vi "PH_Stepmotor_BaseClass.PC set Settings.vi"(0 "i ref in":refnum<vi>, 1 "axis":i32=-1, 2 "Settings to set":T1={"Sign change"=FALSE, "Width"=0.0, "Calibration"=0.0, "Unit"="Steps", "Motor Type"=enum."Unspecific", "Unit Width"="", "Unit CF"=""}, 5 "error in (no error)":errorcluster) -> (14 "i ref out":refnum<vi>, 19 "error out":errorcluster)   [LabVIEW 2014, in "PH_Stepmotor_BaseClass.lvlib"]
doc: "This VI sets - in case of a change - axis settings to own attributes and updates the related DIM service. If necessary, a flag is set."
uses:
  PH_Stepmotor_BaseClass.lvlib
  PH_Stepmotor_BaseClass.Axis Settings.ctl
  PH_Stepmotor_BaseClass.Motor Type.ctl
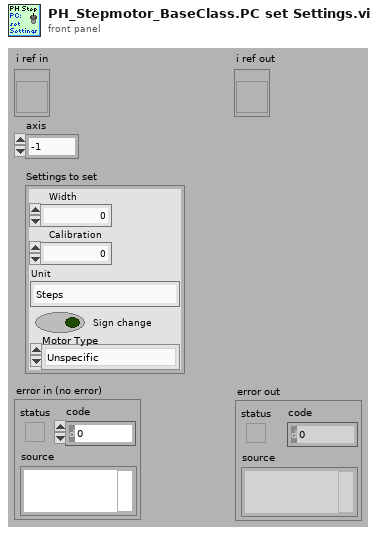
[diagram p1: front panel]
types:
  T1 = typedef "PH_Stepmotor_BaseClass.lvlib/PH_Stepmotor_BaseClass.Axis Settings.ctl" = cluster{"Sign change":bool, "Width":dbl, "Calibration":dbl, "Unit":string, "Motor Type":T2, "Unit Width":string, "Unit CF":string}
  T2 = typedef "PH_Stepmotor_BaseClass.lvlib/PH_Stepmotor_BaseClass.Motor Type.ctl" = enum16{"Unspecific", "OWIS 49.120.2633", "OWIS 49.060.1033", "OWIS 43.040.2558", "Diamond Motion 2200 series", "OWIS 49.120.266B.MV6", "Calorimeter", "Linear Stage 1", "MICOS VT-80", "MICOS VT-80 S", "Standa Rotstage nt0.95A", "PUF RA 320.200", "PUF RA 800.200", "PUF RA 800.400", "PUF RA 400.50", "1324.nn.800.50", "1324.n9c.800.50", "1324.nn.320.200", "1324.nn.400.200", "1324.nn.800.200", "1324.nn.400.50", "1324.8c9c.800.50", "1324.8c9c.400.200"}
  T3 = typedef "PH_Stepmotor_BaseClass.lvlib/PH_Stepmotor_BaseClass.Axis Attributes.ctl" = cluster{"Settings":T1, "Endswitch?":bool, "DIM Service IDs":T4, "Activity":T5, "Configured?":bool, "Position":cluster{"Current":i32, "Target":i32}, "Position to set":cluster{"New?":bool, "Wanted":i32}, "Stop?":bool, "Reset?":bool, "Move?":bool, "Nothing connected?":bool}
  T4 = typedef "PH_Stepmotor_BaseClass.lvlib/PH_Stepmotor_BaseClass.Axis DIM Service IDs.ctl" = cluster{"Settings":i32, "Information":i32}
  T5 = typedef "PH_Stepmotor_BaseClass.lvlib/PH_Stepmotor_BaseClass.Axis Activity.ctl" = enum16{"No Information", "stopped", "running", "Failure", "Alarm", "stopped at backward ES", "stopped at foreward ES"}
  T6 = typedef "PH_Stepmotor_BaseClass.lvlib/PH_Stepmotor_BaseClass.i attribute.ctl" = cluster{"Device Error":errorcluster, "Axes PSDB Thread":cluster{"Ref":refnum<vi>, "Q-Ref":refnum<queue>, "Data Status":T7}, "Axes":T3[], "Axes PSDB Infos":cluster{"GUI Name":string, "PSDB Instance ID":i32, "PSDB Status Service ID":i32, "Axis":i32, "Class":string}[], "GUI Refs":T8}
  T7 = typedef "PH_PSDBWriter.lvlib/PH_PSDBWriter.Data Status.ctl" = i16
  T8 = typedef "PH_Stepmotor_BaseClass.lvlib/PH_Stepmotor_BaseClass.GUI Refs.ctl" = cluster{"Axes Configuration":refnum<vi>, "Device Error":refnum<vi>, "Axes PSDB Infos":refnum<vi>}
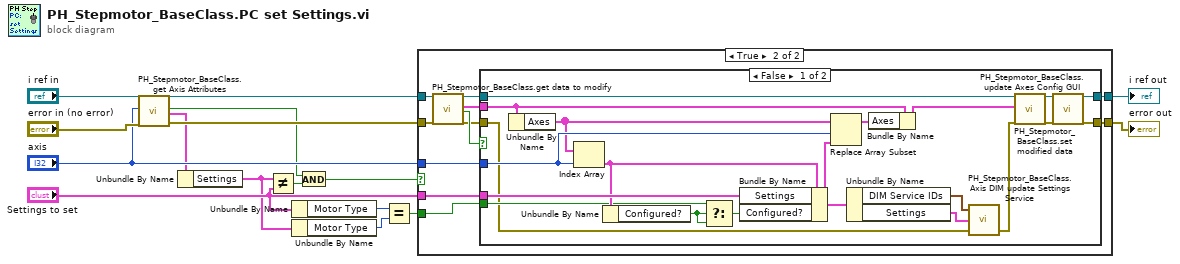
[diagram p0: block diagram]
diagram:
  n1 = call "PH_Stepmotor_BaseClass.get Axis Attributes.vi"("VI in"="i ref in", "Axis"="axis", "error in (no error)"="error in (no error)") -> ("VI out"=w11:refnum<vi>, "Axis found?"=w8:bool, "Axis Attributes"=w9:T3, "error out"=w13:errorcluster)  [unwired: 13 in]
  n2 = Unbundle By Name(w9) -> ("Settings"=w5:T1)
  n3 = Not Equal?(x=w5, y="Settings to set") -> (x != y?=w7:bool)
  n4 = Unbundle By Name("Settings to set") -> ("Motor Type"=w3:T2)
  n5 = Unbundle By Name(w5) -> ("Motor Type"=w2:T2)
  n6 = And(x=w8, y=w7) -> (x .and. y?=w4:bool)
  n7 = Equal?(x=w3, y=w2) -> (x = y?=w1:bool)
  n8 = case shown="True" w4 {
    tunnel: [w18 w25] -> w15
    tunnel: [w17 w24] -> w14
    tunnel: w13 -> [w17 w23]
    tunnel: w11 -> [w18 w22]
    tunnel: "axis" -> [_ w21]
    tunnel: "Settings to set" -> [_ w20]
    tunnel: w1 -> [_ w19]
    frame False {
    }
    frame True {
      n9 = call "PH_Stepmotor_BaseClass.get data to modify.vi"("i ref in"=w22, "error in (no error)"=w23) -> ("i ref out"=w27:refnum<vi>, "i attribute"=w26:T6, "timed out"=w29:bool, "error out"=w28:errorcluster)  [unwired: 14 in]
      n10 = case shown="False" w29 {
        tunnel: [w30 w51] -> w24
        tunnel: w28 -> [w34 w51]
        tunnel: [w31 w50] -> w25
        tunnel: w27 -> [w46 w50]
        tunnel: w26 -> [w49 _]
        tunnel: w21 -> [w45 _]
        tunnel: w20 -> [w42 _]
        tunnel: w19 -> [w36 _]
        frame False {
          n11 = Unbundle By Name(w49) -> ("Axes"=w40:T3[])
          n12 = Index Array(array=w40, index=w45) -> (element=w39:T3)
          n13 = Unbundle By Name(w39) -> ("Configured?"=w38:bool)
          n14 = Select(t=w36, s=w38, f=w38) -> (s? t:f=w37:bool)
          n15 = Bundle By Name(cluster=w39, "Settings"=w42, "Configured?"=w37) -> (w41:T3)
          n16 = Replace Array Subset(array=w40, new element=w41, index=w45) -> (w47:T3[])
          n17 = Unbundle By Name(w41) -> ("DIM Service IDs"=w44:T4, "Settings"=w35:T1)
          n18 = Bundle By Name(cluster=w49, "Axes"=w47) -> (w48:T6)
          n19 = call "PH_Stepmotor_BaseClass.Axis DIM update Settings Service.vi"("error in (no error)"=w34, "Axis Settings"=w35, "Axis DIM IDs"=w44) -> ("error out"=w43:errorcluster)  [unwired: 2 in]
          n20 = call "PH_Stepmotor_BaseClass.set modified data.vi"("i ref in"=w46, "i attribute"=w48, "error in (no error)"=w43) -> ("i ref out"=w32:refnum<vi>, "error out"=w33:errorcluster)  [unwired: 15 in]
          n21 = call "PH_Stepmotor_BaseClass.update Axes Config GUI.vi"("VI in"=w32, "error in (no error)"=w33) -> ("VI out"=w31:refnum<vi>, "error out"=w30:errorcluster)  [unwired: 16 in]
        }
        frame True {
          (unwired) TRUE
        }
      }
    }
  }
  "error out" <- w14
  "i ref out" <- w15
